vi "Datos gita new.vi"() -> ()   [LabVIEW 2017]
panel:
  out "XY Graph 2":cluster{"Y":dbl[], "Y":dbl[]}[](graph) caption="XY Graph"
  in  "Archivo Txt":path
  out "Potencia":dbl
  out "theta":dbl
  in  "Angulo inicial":dbl
  in  "Paso motor":dbl
  out "path":path
  out "concatenated string":string
  in  "Numeric":i32
  out "Reconocimiento 3":T1(plugin-control)
  out "Lectura":string
  out "Imagen orginal 2":T1(plugin-control)
  in  "Dirección donde están las fotos":path
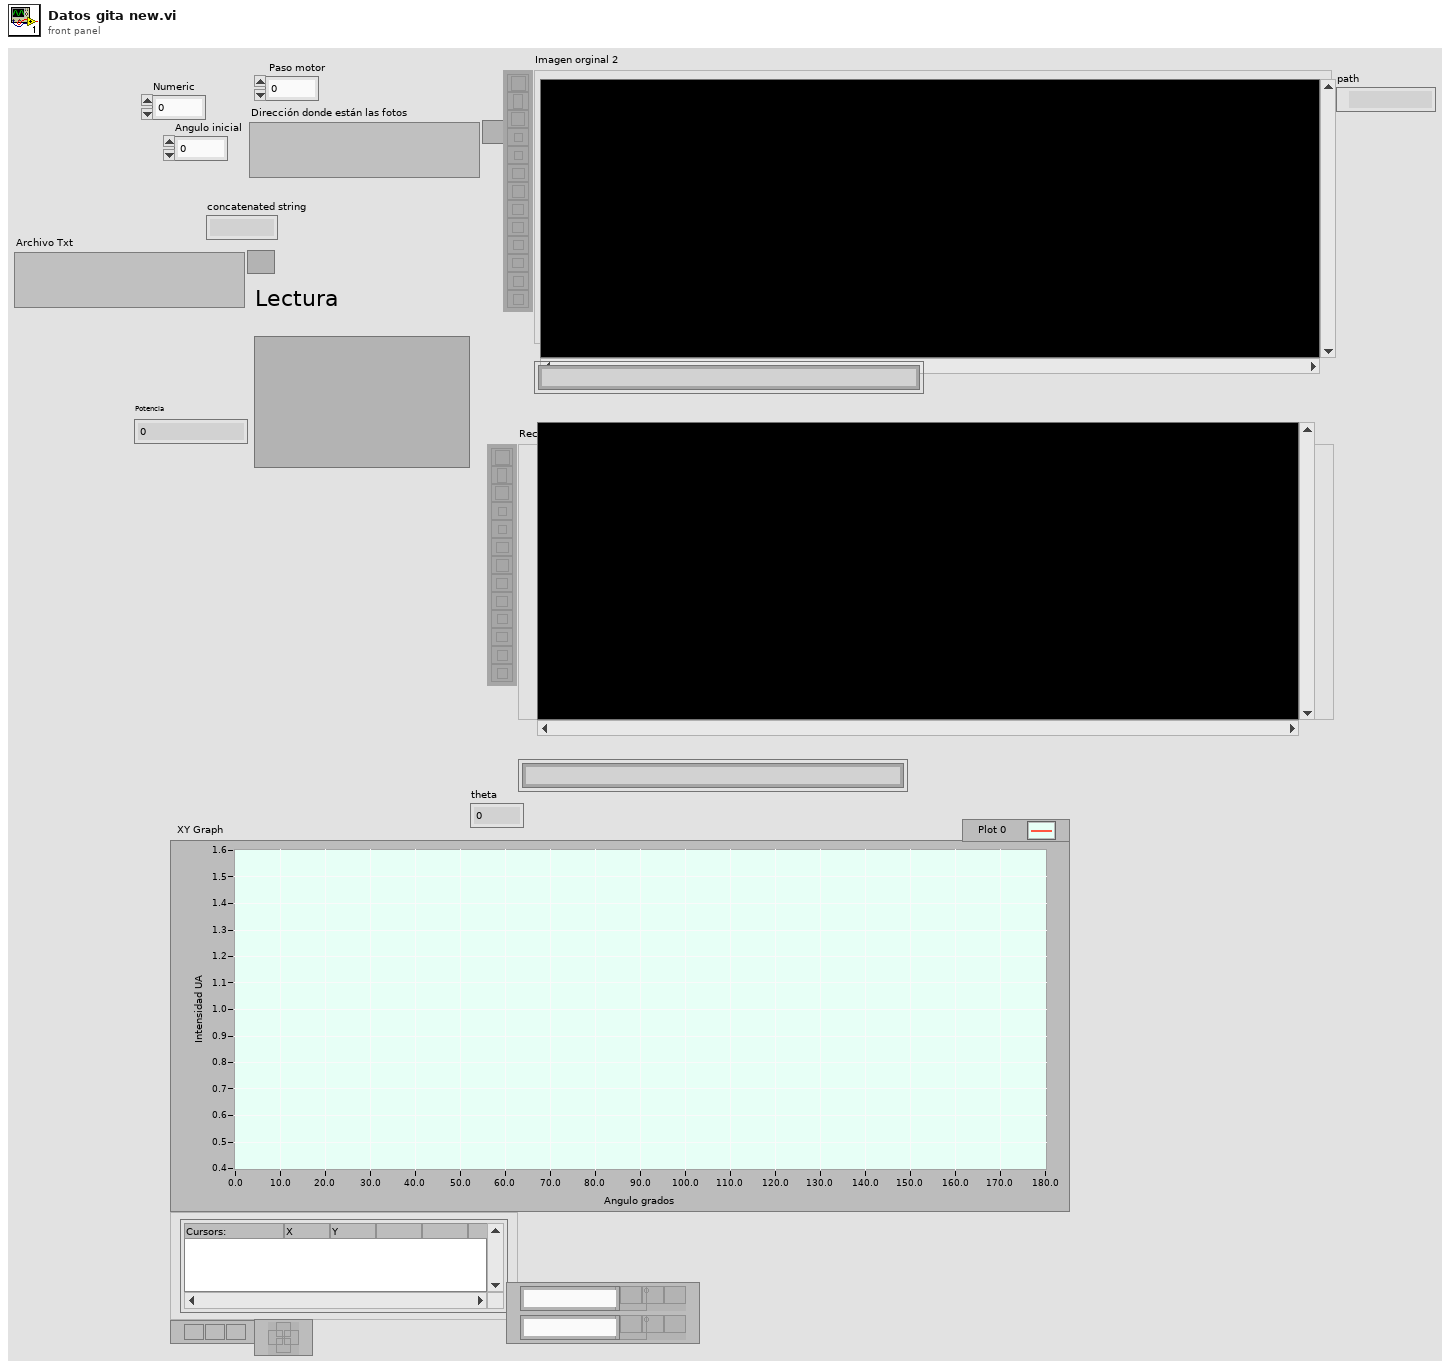
[diagram p1: front panel]
types:
  T1 = typedef "IMAQ Image.ctl" = refnum<image>
  T2 = enum16{"open", "replace", "create", "open or create", "replace or create", "replace or create with confirmation"}
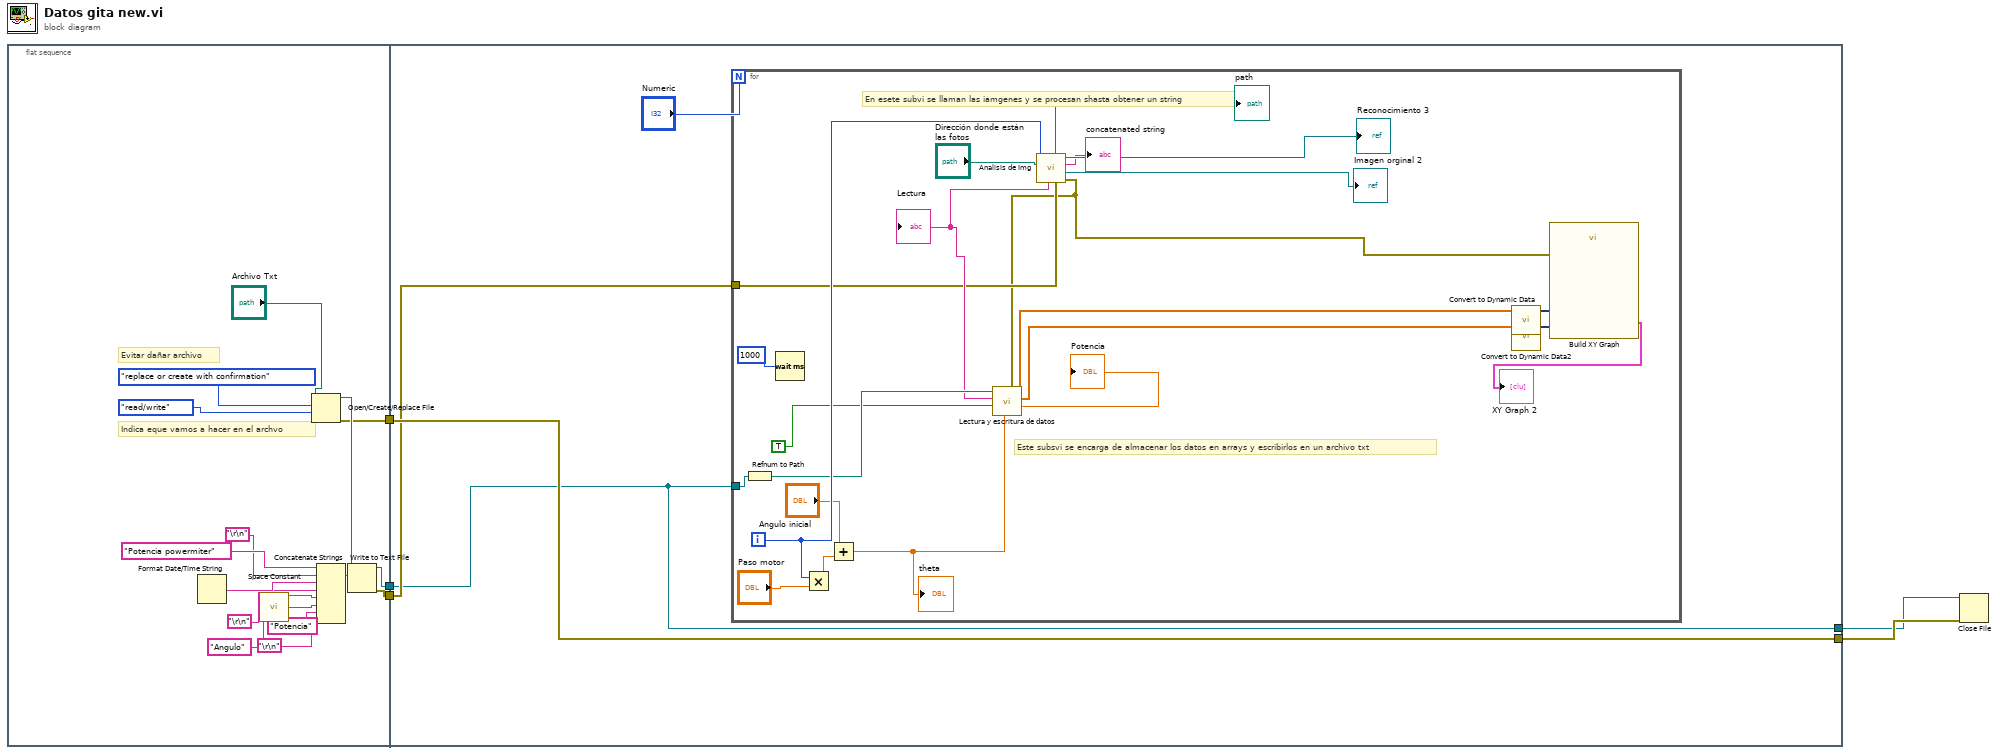
[diagram p0: block diagram]
diagram:
  n1 = flat-sequence {
    tunnel: [w9] -> w5
    tunnel: [w7] -> w4
    tunnel: [w6] -> w3
    tunnel: w5 -> [w22]
    tunnel: [w22] -> w1
    tunnel: [w24] -> w2
    tunnel: w4 -> [w24]
    tunnel: w3 -> [w23]
    frame #0 {
      # "Indica eque vamos a hacer en el archvo"
      # "Evitar dañar archivo"
      n2 = Format Date/Time String() -> (date/time string=w19:string)  [unwired: 3 in]
      n3 = call <vilib>:"Space Constant.vi"() -> ("String"=w21:string)
      n4 = Open/Create/Replace File(file path (use dialog)="Archivo Txt", operation (0:open)=T2."replace or create with confirmation", access (0:read/write)=enum16{"read/write", "read-only", "write-only"}."read/write") -> (refnum out=w12:refnum<file>, error out=w7:errorcluster)  [unwired: 3 in, 1 out]
      n5 = Concatenate Strings("Potencia powermiter", "\r\n", w19, "\r\n", "Angulo", w21, "Potencia", "\r\n") -> (w20:string)
      n6 = Write to Text File(file (use dialog)=w12, text=w20) -> (refnum out=w9:refnum<file>, error out=w6:errorcluster)  [unwired: 2 in, 1 out]
    }
    frame #1 {
      n7 = for {
        N: "Numeric" -> [_]
        tunnel: w22 -> [w26]
        tunnel: w23 -> [w28]
        i -> [w45]
        # "Este subsvi se encarga de almacenar los datos en arrays y escribirlos en un archivo txt"
        # "En esete subvi se llaman las iamgenes y se procesan shasta obtener un string"
        n8 = Refnum to Path(1:w26) -> (0:w41:path)
        n9 = Wait (ms)(milliseconds to wait=u32 1000) -> ()  [unwired: 1 out]
        n10 = Multiply(x=w45, y="Paso motor") -> (x*y=w43:dbl)
        n11 = Add(x="Angulo inicial", y=w43) -> (x+y=w30:dbl)
        "theta" <- w30
        n12 = call "Analisis de Img.vi"("error in"=w28, "File Path in"="Dirección donde están las fotos", "Número de elementos"=w45) -> ("error out"=w27:errorcluster, "Image Out 2"=→"Imagen orginal 2":T1, "concatenated string"=→"concatenated string":string, "Refnum out"=→"Reconocimiento 3":T1, "path"=→"path":path, "Medición"=w29:string)  [unwired: 3 in]
        "Lectura" <- w29
        n13 = call "Lectura y escritura de datos.vi"("error in (no error)"=w27, "Numeric in"=w30, "append to file? (new file:F)"=TRUE, "Medición"=w29, "Path"=w41) -> ("Numeric out"=→"Potencia":dbl, "Array"=w35:dbl[], "Array 2"=w37:dbl[])  [unwired: 4 in]
        n14 = call "Convert to Dynamic Data"("Array"=w37) -> ("Dynamic Data Type"=w36:dynamicdata)  [unwired: 3 in]
        n15 = call "Convert to Dynamic Data2"("Array"=w35) -> ("Dynamic Data Type"=w34:dynamicdata)  [unwired: 3 in]
        n16 = call "Build XY Graph"("error in (no error)"=w27, "Y Input"=w34, "X Input"=w36) -> ("XY Graph"=→"XY Graph 2":cluster{"X":dbl[], "Y":dbl[]}[])  [unwired: 7 in, 1 out]
      }
    }
  }
  n17 = Close File(refnum=w1, error in=w2) -> ()  [unwired: 2 out]
